vi "AdjustLithiumTimings.vi"(9 "Input Trigger Data":T3) -> (3 "Output Trigger Data":T3)   [LabVIEW 2009]
uses:
  Ctrl_Signal.ctl
  Ctrl_Signal_Map.ctl
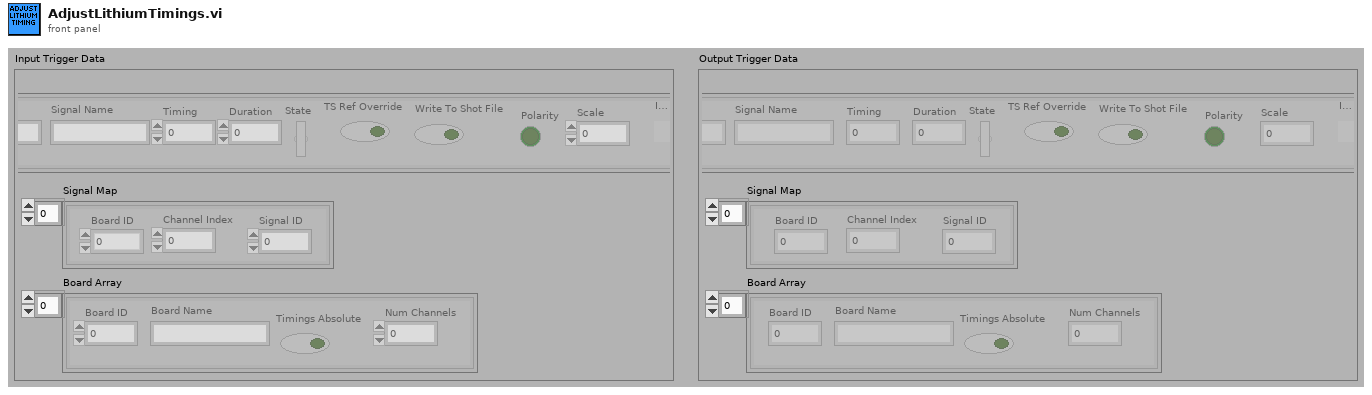
[diagram p1: front panel]
types:
  T1 = typedef "Ctrl_Signal.ctl" = cluster{"Signal Name":string, "Timing":dbl, "Duration":dbl, "State":bool, "TS Ref Override":bool, "Write To Shot File":bool, "Polarity":bool, "Signal ID":dbl, "Scale":dbl, "IsDelay":bool}
  T2 = typedef "Ctrl_Signal_Map.ctl" = cluster{"Channel Index":dbl, "Board ID":dbl, "Signal ID":dbl}
  T3 = cluster{"Signal Array":T1[], "Signal Map":T2[], "Board Array":cluster{"Board ID":dbl, "Board Name":string, "Timings Absolute":bool, "Num Channels":dbl}[]}
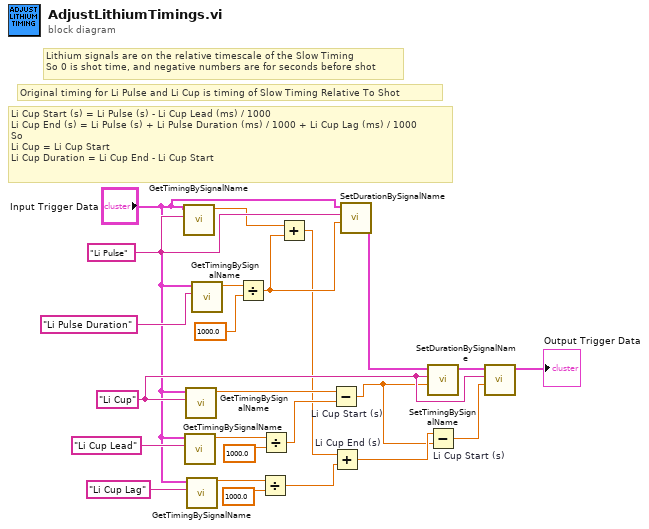
[diagram p0: block diagram]
diagram:
  w19 = "Li Cup" ("Signal Name")
  w8 = "Li Pulse" ("Signal Name")
  # "Original timing for Li Pulse and Li Cup is timing of Slow Timing Relative To Shot"
  # "Lithium signals are on the relative timescale of the Slow Timing\nSo 0 is shot time, and negative numbers are for seconds before shot"
  # "Li Cup Start (s) = Li Pulse (s) - Li Cup Lead (ms) / 1000\nLi Cup End (s) = Li Pulse (s) + Li Pulse Duration (ms) / 1000 + Li Cup Lag (ms) / 1000\nSo\nLi Cup = Li Cup Start\nLi Cup Duration = Li Cup End - Li Cup Start"
  n1 = call "GetTimingBySignalName.vi"("Signal Name"=w8, "Trigger Data"="Input Trigger Data") -> ("Timing"=w7:dbl)  [unwired: 9 in]
  n2 = call "GetTimingBySignalName.vi"("Signal Name"="Li Cup Lead", "Trigger Data"="Input Trigger Data") -> ("Timing"=w18:dbl)  [unwired: 9 in]
  n3 = call "GetTimingBySignalName.vi"("Signal Name"=w19, "Trigger Data"="Input Trigger Data") -> ("Timing"=w10:dbl)  [unwired: 9 in]
  n4 = call "GetTimingBySignalName.vi"("Signal Name"="Li Cup Lag", "Trigger Data"="Input Trigger Data") -> ("Timing"=w14:dbl)  [unwired: 9 in]
  n5 = call "GetTimingBySignalName.vi"("Signal Name"="Li Pulse Duration", "Trigger Data"="Input Trigger Data") -> ("Timing"=w12:dbl)  [unwired: 9 in]
  n6 = Divide(x=w12, y=1000.0) -> (x/y=w6:dbl)
  n7 = Divide(x=w14, y=1000.0) -> (x/y=w13:dbl)
  n8 = Divide(x=w18, y=1000.0) -> (x/y=w16:dbl)
  n9 = Add(x=w7, y=w6) -> (x+y=w5:dbl)
  n10 = Subtract "Li Cup Start (s)"(x=w10, y=w16) -> (x-y=w3:dbl)
  n11 = Add "Li Cup End (s)"(x=w5, y=w13) -> (x+y=w4:dbl)
  n12 = call "SetDurationBySignalName.vi"("Duration"=w6, "Signal Name"=w8, "Trigger Data Input"="Input Trigger Data") -> ("Trigger Data Output"=w21:T3)  [unwired: 8 in]
  n13 = call "SetTimingBySignalName.vi"("Timing"=w3, "Signal Name"=w19, "Trigger Data Input"=w21) -> ("Trigger Data Output"=w20:T3)  [unwired: 8 in]
  n14 = Subtract "Li Cup Start (s)"(x=w4, y=w3) -> (x-y=w2:dbl)
  n15 = call "SetDurationBySignalName.vi"("Duration"=w2, "Signal Name"=w19, "Trigger Data Input"=w20) -> ("Trigger Data Output"=→"Output Trigger Data":T3)  [unwired: 8 in]
